vi "Event Create.vi"(9 "Actor":refnum<class "Actor.lvclass">, 10 "Alias":string, 11 "Event Create in":refnum<class "Event Create.lvclass">) -> (3 "Event Create out":refnum<class "Event Create.lvclass">)   [LabVIEW 2021, in "Event Create.lvlib" / "Event Create.lvclass"]
uses:
  Event Create.lvclass
  Actor/Actor.lvclass
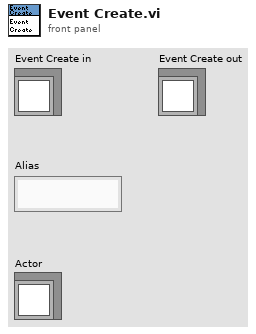
[diagram p1: front panel]
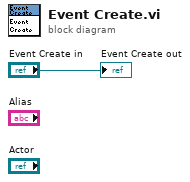
[diagram p0: block diagram]
diagram:
  "Event Create out" <- "Event Create in"
